vi "Write Leakage.vi"(8 "Channel #":i8, 11 "Leakage":dbl) -> ()   [LabVIEW 2020]
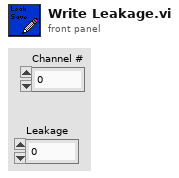
[diagram p1: front panel]
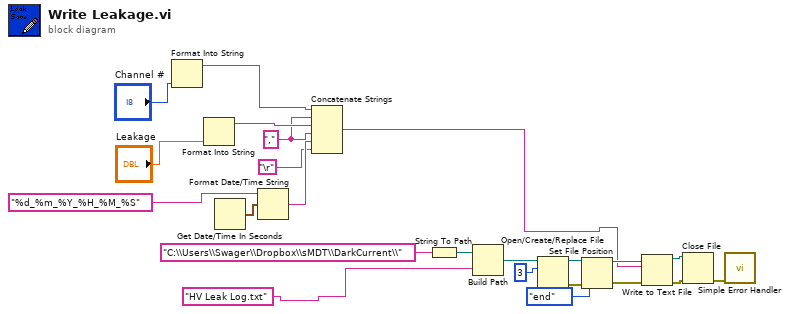
[diagram p0: block diagram]
diagram:
  w2 = ","
  n1 = Format Into String("Channel #") -> (resulting string=w3:string)  [unwired: 3 in, 1 out]
  n2 = Format Into String("Leakage") -> (resulting string=w23:string)  [unwired: 3 in, 1 out]
  n3 = Get Date/Time In Seconds() -> (seconds since 1Jan1904=w16:timestamp)
  n4 = Format Date/Time String(time format string (%c)="%d_%m_%Y_%H_%M_%S", seconds (now)=w16) -> (date/time string=w14:string)  [unwired: 1 in]
  n5 = Concatenate Strings(w3, w2, w23, w2, w14, "\r") -> (w7:string)
  n6 = String To Path(string="C:\\Users\\Swager\\Dropbox\\sMDT\\DarkCurrent\\") -> (path=w17:path)
  n7 = Build Path(base path=w17, name or relative path="HV Leak Log.txt" ("string")) -> (appended path=w18:path)
  n8 = Open/Create/Replace File(file path (use dialog)=w18, operation (0:open)=3) -> (refnum out=w12:refnum<file>, error out=w11:errorcluster)  [unwired: 4 in, 1 out]
  n9 = Set File Position(refnum=w12, from (0:start)=enum16{"start", "end", "current"}."end", error in=w11) -> (refnum out=w9:refnum<file>, error out=w8:errorcluster)  [unwired: 1 in]
  n10 = Write to Text File(file (use dialog)=w9, text=w7, error in=w8) -> (refnum out=w19:refnum<file>, error out=w20:errorcluster)  [unwired: 1 in, 1 out]
  n11 = Close File(refnum=w19, error in=w20) -> (error out=w21:errorcluster)  [unwired: 1 out]
  n12 = call <vilib>:"Simple Error Handler.vi"("error in (no error)"=w21) -> ()  [unwired: 4 in, 5 out]
